vi "RH_PPMU_SetCurrent.vi"(8 "error in":errorcluster, 9 "current level (A)":dbl, 10 "channel list":string, 11 "PPMU Session In":refnum<k15>) -> (0 "error out":errorcluster, 3 "PPMU Session Out":refnum<k15>)   [LabVIEW 2023, in "ResourceHandling.lvlib"]
doc: "Set Current level"
uses:
  ResourceHandling.lvlib
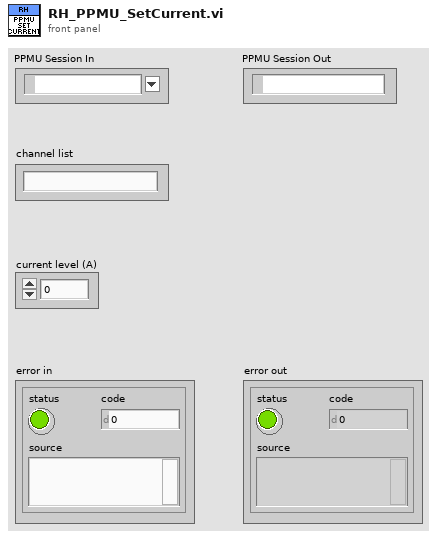
[diagram p1: front panel]
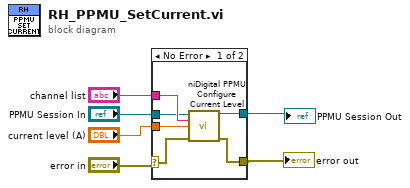
[diagram p0: block diagram]
diagram:
  n1 = case shown="No Error" "error in" {
    selector: "error in" -> [w7 w13]
    tunnel: "channel list" -> [w12 _]
    tunnel: "current level (A)" -> [w11 _]
    tunnel: [w10 w14] -> w4
    tunnel: "PPMU Session In" -> [w9 w14]
    tunnel: [w8 w13] -> w2
    frame No Error {
      n2 = call <instrlib>:"niDigital PPMU Configure Current Level.vi"("instrument handle"=w9, "channel list"=w12, "current level (A)"=w11, "error in"=w7) -> ("instrument handle out"=w10:refnum<k15>, "error out"=w8:errorcluster)  [unwired: 10 in]
    }
    frame Error {
    }
  }
  "PPMU Session Out" <- w4
  "error out" <- w2
